vi "1.1 Steering Controls With Lead Compensator.vi"(4 "Steering Integer Setpoint":i32) -> ()   [LabVIEW 2010]
uses:
  1.0-Hindbrain Global.vi
panel:
  out "Output":fxp<+/-,20,5> format="%.17g"
  in  "Input K s14fxp-6":fxp<+/-,14,-6>
  in  "Input C u8fxp-2":fxp<+/-,17,17>
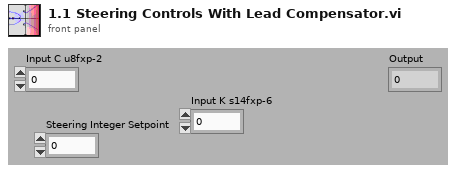
[diagram p1: front panel]
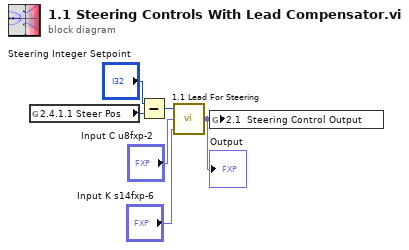
[diagram p0: block diagram]
diagram:
  n1 = global read "1.0-Hindbrain Global.vi" "2.4.1.1 Steer Pos"() -> (w5:i32)
  n2 = Subtract(x="Steering Integer Setpoint", y=w5) -> (x-y=w4:i32)
  n3 = call "1.1 Lead For Steering.vi"("Input K s14fxp-6"="Input K s14fxp-6", "Input C u8fxp-2"="Input C u8fxp-2", "Error Input"=w4) -> ("Controls Output"=w1:fxp<+/-,20,5>)
  "Output" <- w1
  n4 = global write "1.0-Hindbrain Global.vi" "2.1  Steering Control Output"(w1) -> ()
